vi "ConnectWifi.vi"(8 "error in":errorcluster, 10 "Password":string="88888888", 11 "WIFIName":string="Honor V10") -> (0 "error out":errorcluster caption="错误输出", 1 "Time":u32, 2 "TotalOut":string, 3 "Acess":bool)   [LabVIEW 2013]
uses:
  <vilib>/Utility/sysdir.llb/System Directory Type.ctl
panel:
  in  "配置连接次数":i32=5
  out "stdout_Add":string caption="标准输出"
  out "stdout_Connect":string caption="标准输出"
  in  "Delay Time":dbl=1.0 caption="ConfigTime"
  out "新文本":string
  out "原文本":string
  out "数值":i32
  out "SD":path caption="系统目录"
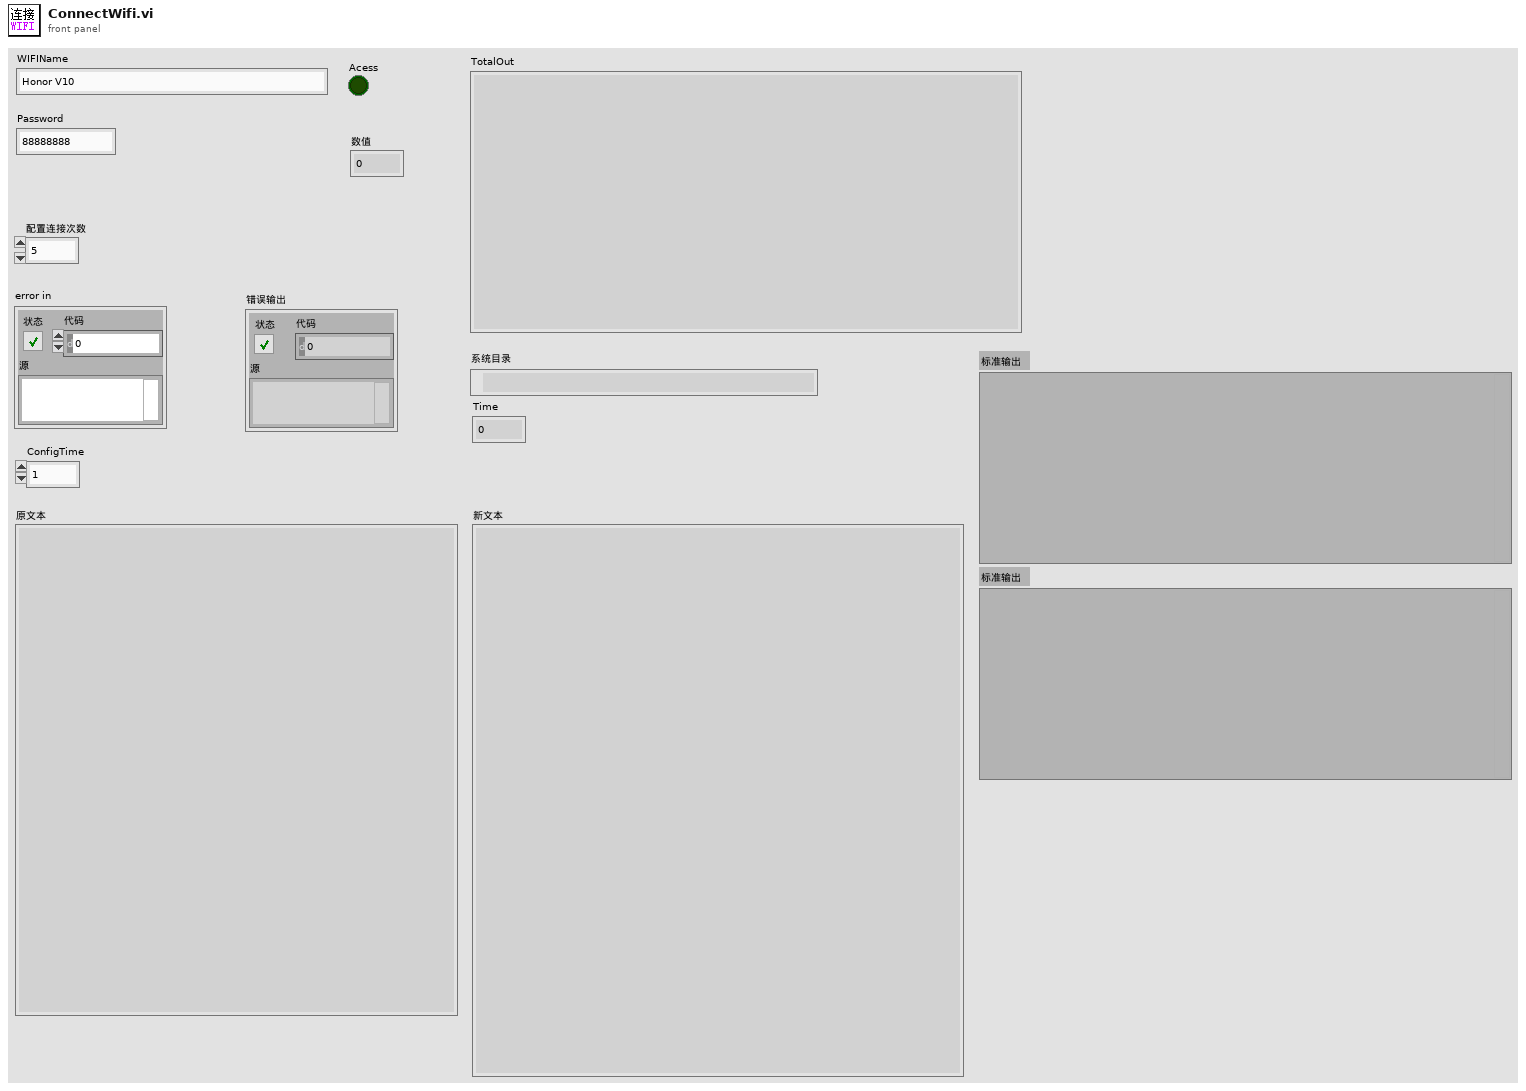
[diagram p1: front panel]
types:
  T1 = typedef "System Directory Type.ctl" = i32
  T2 = enum16{"open", "replace", "create", "open or create", "replace or create", "replace or create with confirmation"}
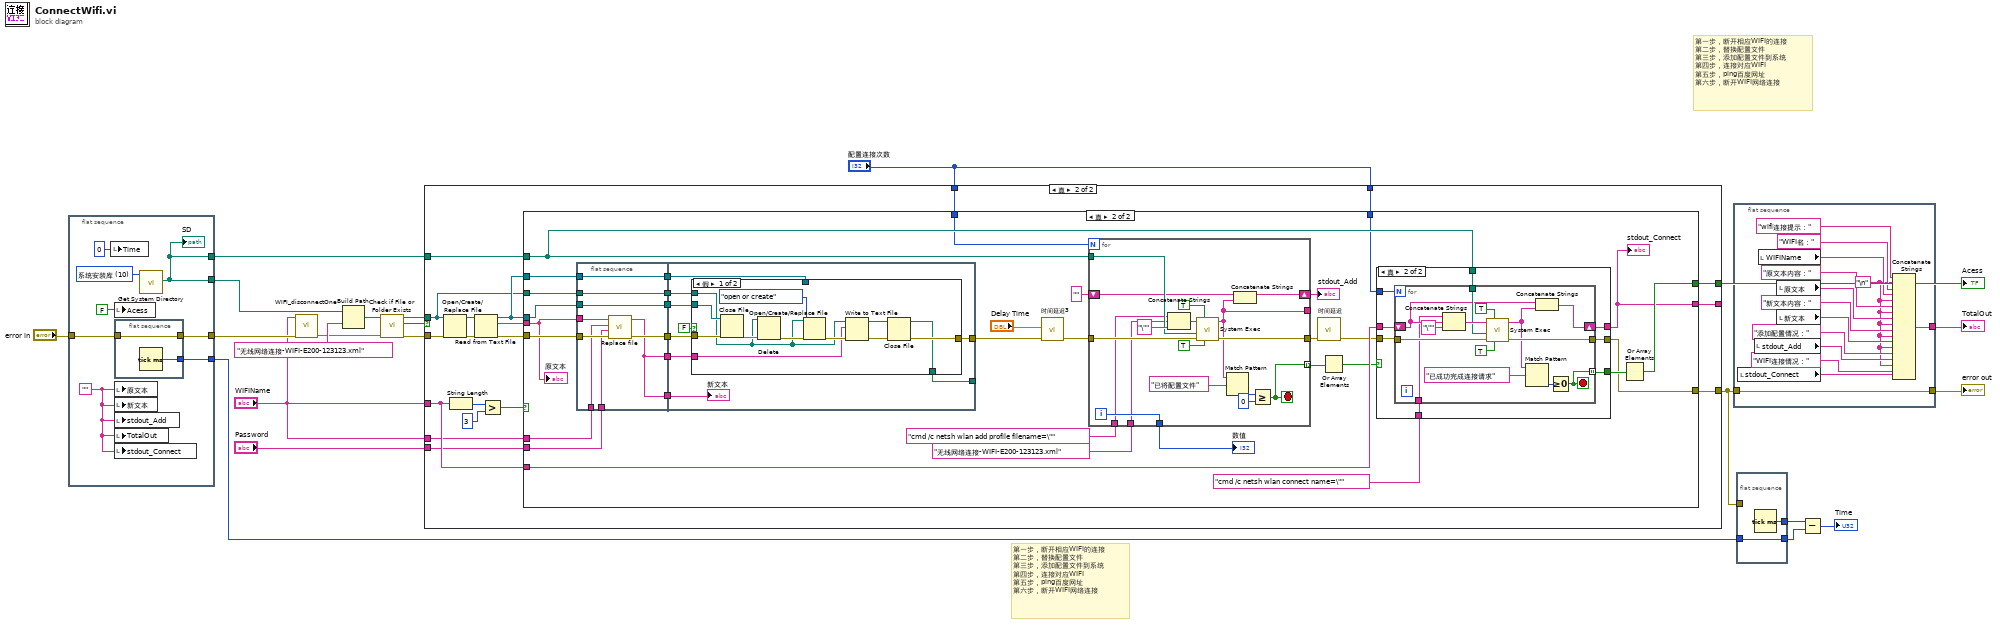
[diagram p0: block diagram]
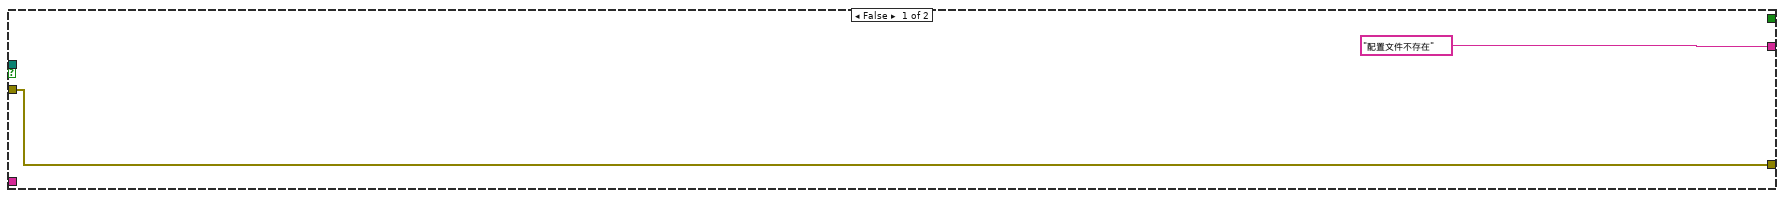
[diagram p2: hidden frame]
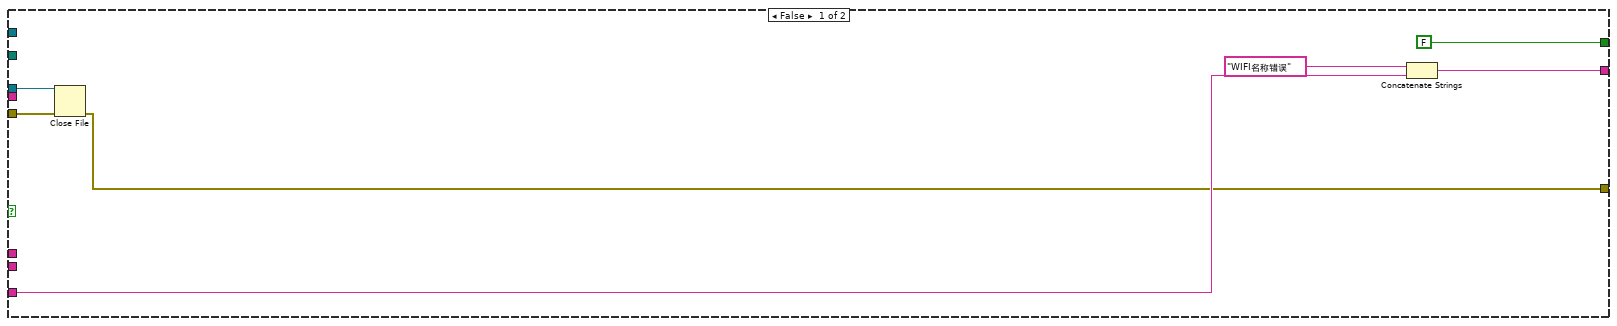
[diagram p3: hidden frame]
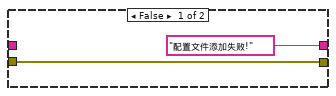
[diagram p4: hidden frame]
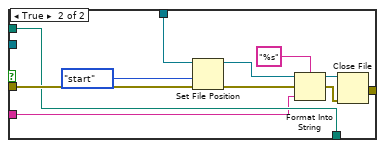
[diagram p5: hidden frame]
diagram:
  # "第一步，断开相应WIFI的连接\n第二步，替换配置文件\n第三步，添加配置文件到系统\n第四步，连接对应WIFI\n第五步，ping百度网址\n第六步，断开WIFI网络连接"
  # "第一步，断开相应WIFI的连接\n第二步，替换配置文件\n第三步，添加配置文件到系统\n第四步，连接对应WIFI\n第五步，ping百度网址\n第六步，断开WIFI网络连接"
  n1 = flat-sequence {
    tunnel: [w28] -> w18
    tunnel: [w28] -> w16
    tunnel: "error in" -> [w25]
    tunnel: [w26] -> w6
    tunnel: [w24] -> w11
    frame #0 {
      w27 = ""
      w29 = T1 10 items=["用户目录"=0, "用户桌面"=1, "用户文档"=2, "用户应用程序数据"=3, "用户设置"=4, "用户临时目录"=5, "公共文档"=6, "公共应用程序数据"=7, "公共设置"=8, "公共缓存"=13, "系统核心库"=9, "系统安装库"=10, "应用程序文件"=11, "启动盘根目录"=12] ("system directory type")
      n2 = local write "Time"(u32 0 ("Time")) -> ()
      n3 = local write "Acess"(FALSE ("Acess")) -> ()
      n4 = flat-sequence {
        tunnel: [w31] -> w26
        tunnel: w25 -> [w31]
        tunnel: [w30] -> w24
        frame #0 {
          n5 = Tick Count (ms)() -> (millisecond timer value=w30:u32)
        }
      }
      n6 = local write "原文本"(w27) -> ()
      n7 = local write "新文本"(w27) -> ()
      n8 = local write "stdout_Add"(w27) -> ()
      n9 = local write "TotalOut"(w27) -> ()
      n10 = local write "stdout_Connect"(w27) -> ()
      n11 = call <vilib>:"Get System Directory.vi"("system directory type"=w29) -> ("system directory"=w28:path)  [unwired: 10 in]
      "SD" <- w28
    }
  }
  n12 = call "WIFI_disconnectOne.vi"("错误输入"=w6, "WIFI_Name"="WIFIName") -> ("error out"=w7:errorcluster)  [unwired: 8 in, 1 out]
  n13 = Build Path(base path=w18, name or relative path="无线网络连接-WIFI-E200-123123.xml" ("名称或相对路径")) -> (appended path=w21:path)
  n14 = call <vilib>:"Check if File or Folder Exists.vi"("error in (no error)"=w7, "path"=w21) -> ("error out"=w19:errorcluster, "file or folder exists?"=w14:bool, "dup path"=w15:path)  [unwired: 7 in]
  n15 = case shown="真" w14 {
    tunnel: w19 -> [w32 w49]
    tunnel: w16 -> [_ w47]
    tunnel: "WIFIName" -> [_ w46]
    tunnel: [_ w44] -> w4
    tunnel: ["配置文件不存在" ("standard output") w43] -> _
    tunnel: [w32 w39] -> w1
    tunnel: w15 -> [_ w38]
    tunnel: "Password" -> [_ w37]
    tunnel: "WIFIName" -> [_ w36]
    tunnel: "配置连接次数" -> [_ w35]
    tunnel: "配置连接次数" -> [_ w34]
    frame False {
    }
    frame True {
      n16 = Open/Create/Replace File(file path (use dialog)=w38, error in=w49) -> (refnum out=w52:refnum<file>, error out=w51:errorcluster)  [unwired: 4 in, 1 out]
      n17 = String Length(string=w46) -> (length=w42:i32)
      n18 = Read from Text File(file (use dialog)=w52, error in=w51) -> (refnum out=w45:refnum<file>, text=w48:string, error out=w50:errorcluster)  [unwired: 2 in, 1 out]
      n19 = Greater?(x=w42, y=3) -> (0:w40:bool)
      n20 = case shown="真" w40 {
        tunnel: w50 -> [w58 w81]
        tunnel: w45 -> [_ w92]
        tunnel: w48 -> [_ w76]
        tunnel: w46 -> [w57 w90]
        tunnel: w47 -> [_ w89]
        tunnel: w45 -> [w59 w87]
        tunnel: [w53 w65] -> w39
        tunnel: [FALSE ("Acess") w68] -> w44
        tunnel: [w55 w67] -> w43
        tunnel: w38 -> [_ w88]
        tunnel: w37 -> [_ w78]
        tunnel: w36 -> [_ w77]
        tunnel: w35 -> [_ w73]
        tunnel: w34 -> [_ w72]
        frame False {
          n21 = Close File(refnum=w59, error in=w58) -> (error out=w53:errorcluster)  [unwired: 1 out]
          n22 = Concatenate Strings("WIFI名称错误" ("字符串"), w57) -> (w55:string)
        }
        frame True {
          n23 = flat-sequence {
            tunnel: w87 -> [w141]
            tunnel: w88 -> [w142]
            tunnel: w92 -> [w143]
            tunnel: [w143] -> w84
            tunnel: [w142] -> w83
            tunnel: [w141] -> w82
            tunnel: w81 -> [w140]
            tunnel: [w139] -> w80
            tunnel: [w135] -> w79
            tunnel: w78 -> [w138]
            tunnel: w77 -> [w137]
            tunnel: w76 -> [w136]
            tunnel: [w135] -> w66
            tunnel: [w152] -> w93
            tunnel: [w147] -> _
            tunnel: w84 -> [w151]
            tunnel: w83 -> [w149]
            tunnel: w82 -> [w148]
            tunnel: w80 -> [w146]
            tunnel: w79 -> [w145]
            tunnel: w66 -> [w144]
            frame #0 {
              n24 = call "Replace file.vi"("error in"=w140, "password"=w138, "new wifi name"=w137, "txt input"=w136) -> ("error out"=w139:errorcluster, "txt output"=w135:string)  [unwired: 6 in]
            }
            frame #1 {
              n25 = case shown="假" FALSE {
                tunnel: [w156 w170] -> w152
                tunnel: w146 -> [w163 w169]
                tunnel: w151 -> [_ w168]
                tunnel: w149 -> [w155 w166]
                tunnel: w148 -> [w164 _]
                tunnel: [w154 w166] -> w147
                tunnel: w145 -> [w153 w165]
                frame False {
                  n26 = Close File(refnum=w164, error in=w163) -> (error out=w162:errorcluster)  [unwired: 1 out]
                  n27 = Delete(path (use dialog)=w155, error in=w162) -> (error out=w160:errorcluster)  [unwired: 3 in, 2 out]
                  n28 = Open/Create/Replace File(file path (use dialog)=w155, error in=w160, operation (0:open)=T2."open or create" ("操作(0:open)")) -> (error out=w159:errorcluster)  [unwired: 3 in, 2 out]
                  n29 = Write to Text File(file (use dialog)=w155, text=w153, error in=w159) -> (refnum out=w158:refnum<file>, error out=w157:errorcluster)  [unwired: 1 in, 1 out]
                  n30 = Close File(refnum=w158, error in=w157) -> (path=w154:path, error out=w156:errorcluster)
                }
                frame True {
                  n31 = Set File Position(refnum=w168, from (0:start)=enum16{"start", "end", "current"}."start" ("自（0:起始）"), error in=w169) -> (refnum out=w171:refnum<file>, error out=w174:errorcluster)  [unwired: 1 in]
                  n32 = Format Into String(format string="%s" ("格式字符串"), initial string=w171, error in=w174, w165) -> (resulting string=w167:refnum<file>, error out=w173:errorcluster)
                  n33 = Close File(refnum=w167, error in=w173) -> (error out=w170:errorcluster)  [unwired: 1 out]
                }
              }
              "新文本" <- w144
            }
          }
          n34 = call "时间延迟3"("error in (no error)"=w93, "Delay Time (s)"="Delay Time") -> ("error out"=w86:errorcluster)  [unwired: 9 in]
          n35 = for {
            N: w73 -> [_]
            tunnel: [w130] -> w91
            tunnel: w89 -> [w129]
            tunnel: w86 -> [w128]
            shift-right: [w126] -> w74
            shift-left: "" -> [w127]
            tunnel: [w125] -> _
            tunnel: [w121] -> w61 mode=indexing
            tunnel: [w120] -> w71
            tunnel: "cmd /c netsh wlan add profile filename=\"" ("command line") -> [w119]
            tunnel: "无线网络连接-WIFI-E200-123123.xml" ("名称或相对路径") -> [w118]
            i -> [w120]
            stop <- w121 stop-if-true
            n36 = Concatenate Strings(w119, w118, "\"" ("字符串")) -> (w132:string)
            n37 = call <vilib>:"System Exec.vi"("run minimized? (F)"=TRUE, "wait until completion? (T)"=TRUE, "error in (no error)"=w128, "working directory"=w129, "command line"=w132) -> ("error out"=w130:errorcluster, "standard output"=w125:string)  [unwired: 3 in, 2 out]
            n38 = Match Pattern(string=w125, regular expression="已将配置文件") -> (offset past match=w123:i32)  [unwired: 1 in, 3 out]
            n39 = Concatenate Strings(w127, w125) -> (w126:string)
            n40 = Greater Or Equal?(x=w123, y=0) -> (x >= y?=w121:bool)
          }
          "stdout_Add" <- w74
          "数值" <- w71
          n41 = call "时间延迟"("error in (no error)"=w91) -> ("error out"=w70:errorcluster)  [unwired: 10 in]
          n42 = Or Array Elements(Boolean array=w61) -> (logical OR=w60:bool)
          n43 = case shown="真" w60 {
            tunnel: w90 -> [_ w103]
            tunnel: w89 -> [_ w102]
            tunnel: w72 -> [_ w101]
            tunnel: w70 -> [w95 w100]
            tunnel: [_ w99] -> w69
            tunnel: ["配置文件添加失败!" w98] -> w67
            tunnel: [w95 w97] -> w65
            tunnel: "cmd /c netsh wlan connect name=\"" ("command line") -> [_ w96]
            frame False {
            }
            frame True {
              n44 = for {
                N: w101 -> [_]
                tunnel: [w115] -> w97
                tunnel: w102 -> [w112]
                tunnel: w100 -> [w111]
                shift-right: [w110] -> w98
                shift-left: w103 -> [w109]
                tunnel: [w105] -> w99 mode=indexing
                tunnel: w96 -> [w104]
                stop <- w105 stop-if-true
                n45 = Concatenate Strings(w104, w109, "\"" ("字符串")) -> (w113:string)
                n46 = call <vilib>:"System Exec.vi"("run minimized? (F)"=TRUE, "wait until completion? (T)"=TRUE, "error in (no error)"=w111, "working directory"=w112, "command line"=w113) -> ("error out"=w115:errorcluster, "standard output"=w108:string)  [unwired: 3 in, 2 out]
                n47 = Match Pattern(string=w108, regular expression="已成功完成连接请求") -> (offset past match=w106:i32)  [unwired: 1 in, 3 out]
                n48 = Concatenate Strings(w109, w108) -> (w110:string)
                n49 = Greater Or Equal To 0?(x=w106) -> (x >= 0?=w105:bool)
              }
            }
          }
          "stdout_Connect" <- w67
          n50 = Or Array Elements(Boolean array=w69) -> (logical OR=w68:bool)
          "原文本" <- w76
        }
      }
    }
  }
  "Acess" <- w4
  n51 = flat-sequence {
    tunnel: w1 -> [w189]
    tunnel: [w189] -> w3
    tunnel: [w176] -> w2
    frame #0 {
      w179 = "\n"
      n52 = local read "stdout_Connect"() -> (w177:string)
      n53 = local read "stdout_Add"() -> (w180:string)
      n54 = local read "WIFIName"() -> (w186:string)
      n55 = local read "原文本"() -> (w184:string)
      n56 = local read "新文本"() -> (w182:string)
      n57 = Concatenate Strings("wifi连接提示：", w179, "WIFI名：", w186, w179, "原文本内容：", w179, w184, w179, "新文本内容：", w179, w182, w179, "添加配置情况：", w180, w179, "WIFI连接情况：", w177) -> (w176:string)
    }
  }
  n58 = flat-sequence {
    tunnel: w11 -> [w190]
    tunnel: [w191] -> w10
    tunnel: [w190] -> w9
    tunnel: w1 -> [_]
    frame #0 {
      n59 = Tick Count (ms)() -> (millisecond timer value=w191:u32)
    }
  }
  n60 = Subtract(x=w10, y=w9) -> (x-y=→"Time":u32)
  "TotalOut" <- w2
  "error out" <- w3
